vi "OutputCompressor.vi"   [LabVIEW 2020]
doc: "This VI sends commands to the compressor."
uses:
  GlobalMiscellaneous.vi
  GRNF_Compressor.vi
  <vilib>/Rock Robotics/WPI/Compressor/WPI_CompressorFeedbackMode.ctl
  TAI_Solenoid.vi
types:
  T1 = typedef "WPI_CompressorFeedbackMode.ctl" = enum16{"Analog Only", "Digital Only", "Hybrid"}
  T2 = cluster{"Feedback Sensor":T1, "Max Pressure (PSI)":dbl, "Min Pressure (PSI)":dbl}
  T3 = typedef "WPI_CompressorDevRef.ctl" = cluster{"DevStatus":errorcluster, "Pneumatics Control Module":u8}
  T4 = enum16{"No Changed Output", "New Normal Output", "New Testing Output"}
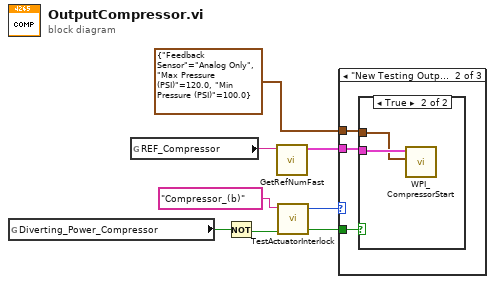
[diagram p0: block diagram]
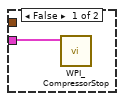
[diagram p3: hidden frame]
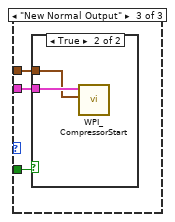
[diagram p4: hidden frame]
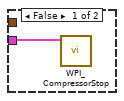
[diagram p5: hidden frame]
diagram:
  n1 = global read "GlobalMiscellaneous.vi" "Diverting_Power_Compressor"() -> (w8:bool)
  n2 = global read "GlobalMiscellaneous.vi" "REF_Compressor"() -> (w1:string)
  n3 = Not(x=w8) -> (.not. x?=w3:bool)
  n4 = call-poly "GetRefNumFast.vi"("RefNum Name"=w1) -> ("Device Reference"=w5:T3)  [unwired: 5 in, 1 out]
  n5 = call-poly "TestActuatorInterlock.vi"("Normal Output"=w3, "Actuator Name"="Compressor_(b)") -> ("Interlocked Output"=w2:bool, "Output Mode"=w6:T4)  [unwired: 3 in]
  n6 = case shown="\"New Testing Output\"" w6 {
    tunnel: w5 -> [_ w11 w17]
    tunnel: w2 -> [_ w9 w16]
    tunnel: T2 {"Feedback Sensor"=enum."Analog Only", "Max Pressure (PSI)"=120.0, "Min Pressure (PSI)"=100.0} ("Feedback Configuration") -> [_ w10 w15]
    frame "No Changed Output", Default {
    }
    frame "New Testing Output" {
      n7 = case shown="True" w9 {
        tunnel: w11 -> [w12 w14]
        tunnel: w10 -> [_ w13]
        frame False {
          n8 = call <vilib>:"WPI_CompressorStop.vi"("CompressorDevRef"=w12) -> ()  [unwired: 9 in, 2 out]
        }
        frame True {
          n9 = call <vilib>:"WPI_CompressorStart.vi"("Feedback Configuration"=w13, "CompressorDevRef"=w14) -> ()  [unwired: 8 in, 2 out]
        }
      }
    }
    frame "New Normal Output" {
      n10 = case shown="True" w16 {
        tunnel: w17 -> [w18 w20]
        tunnel: w15 -> [_ w19]
        frame False {
          n11 = call <vilib>:"WPI_CompressorStop.vi"("CompressorDevRef"=w18) -> ()  [unwired: 9 in, 2 out]
        }
        frame True {
          n12 = call <vilib>:"WPI_CompressorStart.vi"("Feedback Configuration"=w19, "CompressorDevRef"=w20) -> ()  [unwired: 8 in, 2 out]
        }
      }
    }
  }
